vi "TCP Close Client.vi"(8 "error in (no error)":errorcluster, 11 "connection ID":refnum<k5>) -> (0 "error out":errorcluster)   [LabVIEW 2016, in "SLL Easy API via TCP.lvclass"]
doc: "Closes the TCP Connection."
uses:
  SLL Easy API via TCP.lvclass
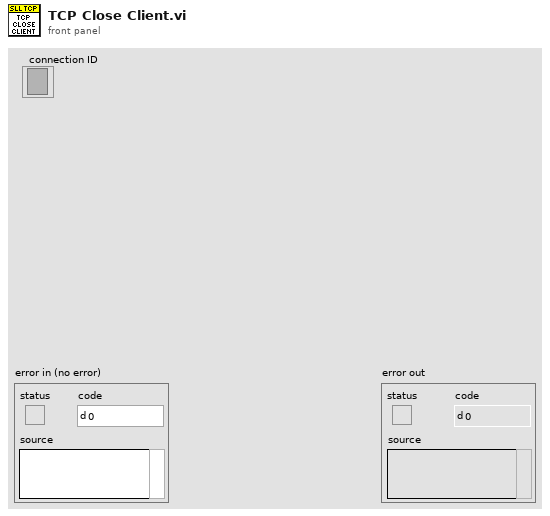
[diagram p1: front panel]
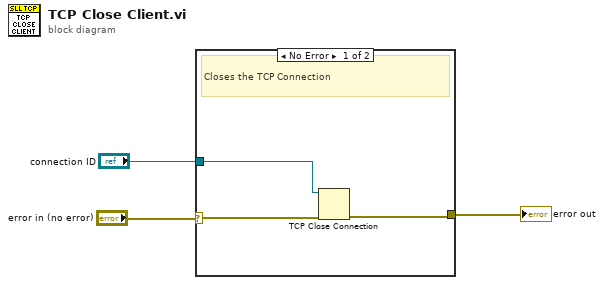
[diagram p0: block diagram]
diagram:
  n1 = case shown="No Error" "error in (no error)" {
    selector: "error in (no error)" -> [w6 w7]
    tunnel: [w5 w7] -> w2
    tunnel: "connection ID" -> [w4 _]
    frame No Error {
      # "Closes the TCP Connection"
      n2 = TCP Close Connection(connection ID=w4, error in (no error)=w6) -> (error out=w5:errorcluster)  [unwired: 1 in, 1 out]
    }
    frame Error {
    }
  }
  "error out" <- w2
